vi "Load_Window_Bounds.vi"(4 "Open at mouse position?":bool, 5 "Open maximised?":bool, 6 "Re-entrant user message window? (F)":bool, 7 "Window Name (i.e. Key)":string, 8 "error in":errorcluster, 9 "Disable":bool, 10 "First Call":bool, 11 "Window VI's Ref":refnum<vi>) -> (0 "error out":errorcluster, 1 "Front Panel.WinBounds":T1, 2 "Window size":cluster{"Horisontal":i16, "Vertical":i16}, 3 "reference out":refnum<vi>)   [LabVIEW 2013]
uses:
  <vilib>/Utility/miscctls.llb/LVRectTypeDef.ctl
  Typedefs/Which path.ctl
  Typedefs/Window position FG states.ctl
  <vilib>/Utility/config.llb/Read Key (String).vi
  <vilib>/Utility/config.llb/NI_LVConfig.lvlib
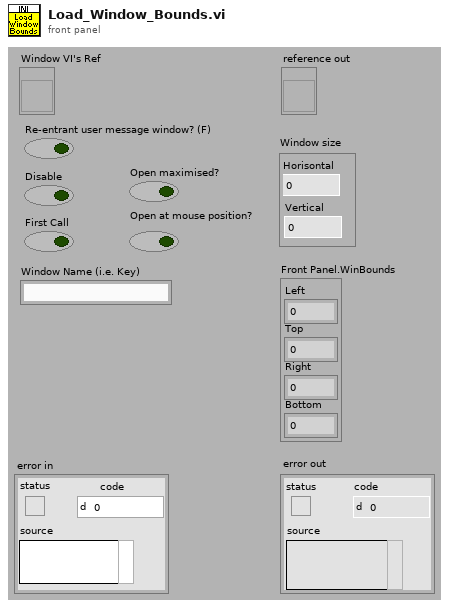
[diagram p1: front panel]
types:
  T1 = typedef "LVRectTypeDef.ctl" = cluster{"Left":i16, "Top":i16, "Right":i16, "Bottom":i16}
  T2 = enum32{"Invalid", "Standard", "Closed", "Hidden", "Minimized", "Maximized"}
  T3 = typedef "Which path.ctl" = enum16{"Configuration Files", "Calibration Files", "Images", "Setup.ini", "Loaded User profile.ini", "User's-Previous session.ini", "New user profile.ini", "Selected User profile.ini", "User profiles folder", "Power meter scaling.txt", "FOV Cal.ini"}
  T4 = typedef "Window position FG states.ctl" = enum16{"Manage", "Query", "Write"}
  T5 = typedef "NI_LVConfig.lvlib/Config Data RefNum.ctl" = refnum<k1>
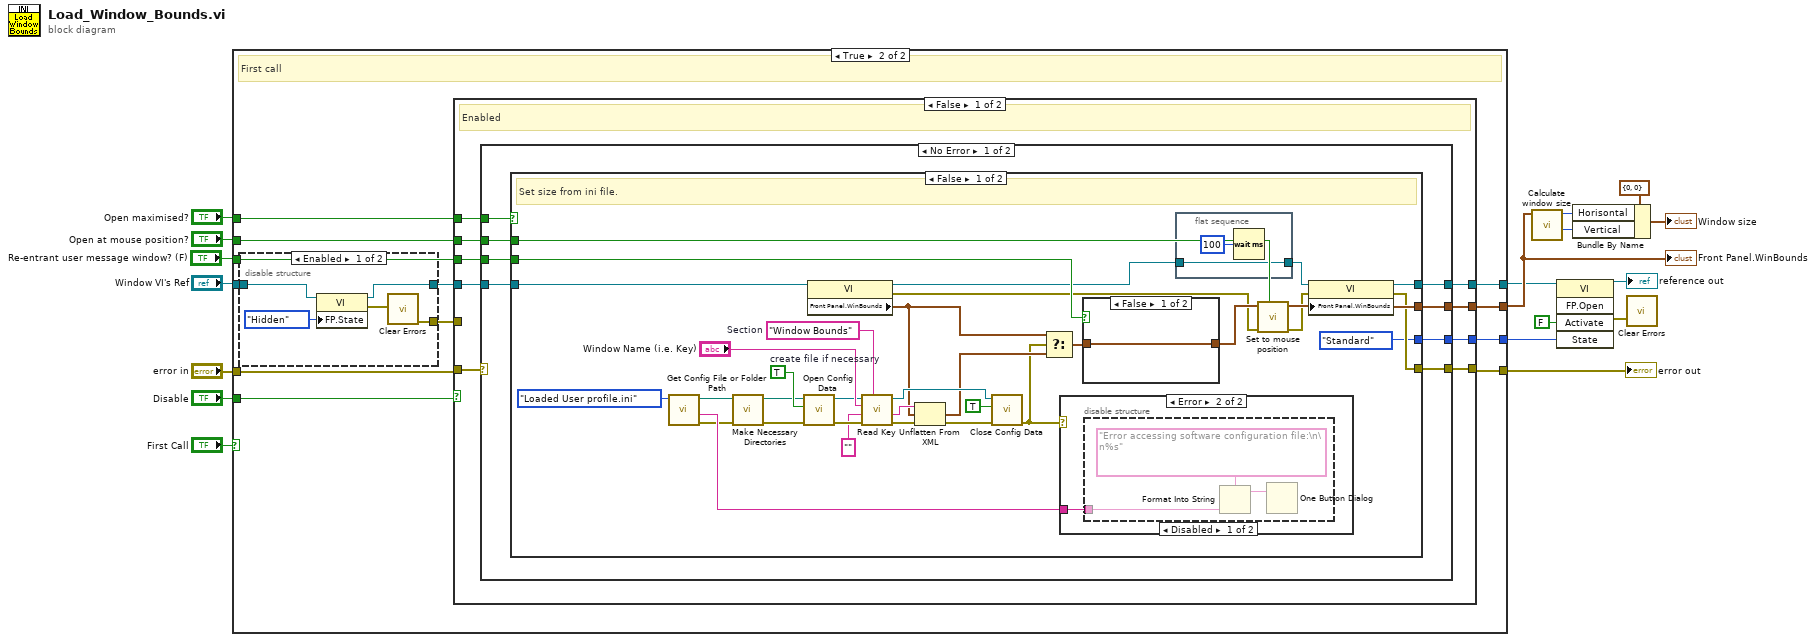
[diagram p0: block diagram]
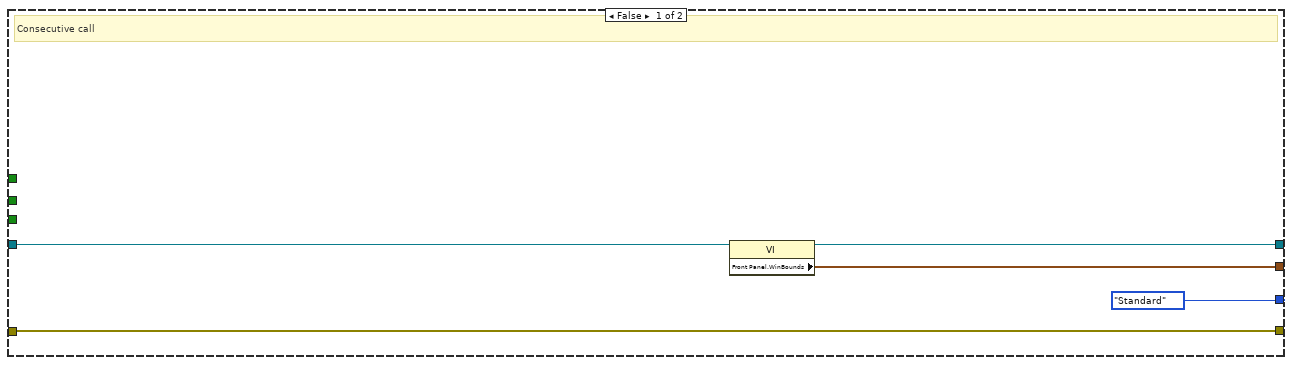
[diagram p2: hidden frame]
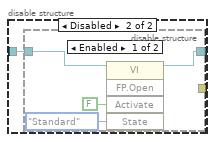
[diagram p3: hidden frame]
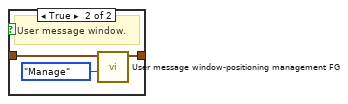
[diagram p5: hidden frame]
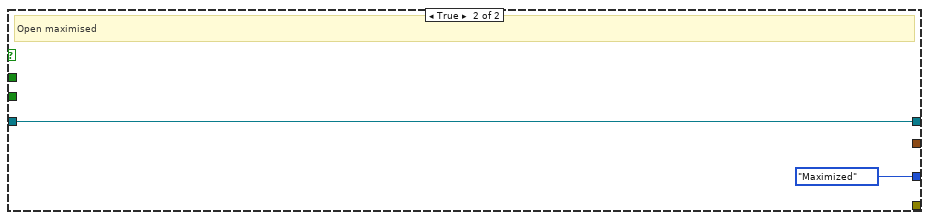
[diagram p8: hidden frame]
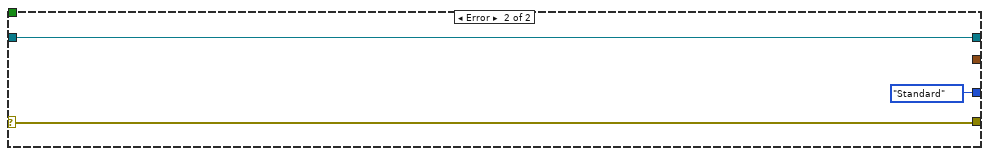
[diagram p9: hidden frame]
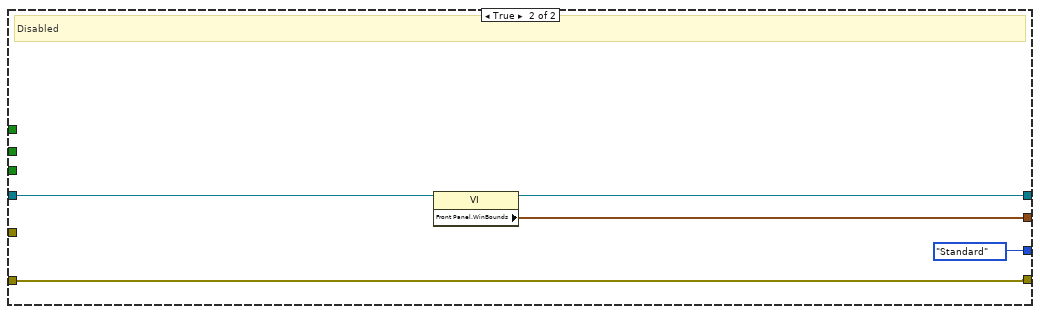
[diagram p10: hidden frame]
diagram:
  n1 = case shown="True" "First Call" {
    tunnel: "error in" -> [w23 w35]
    tunnel: "Disable" -> [_ w34]
    tunnel: "Window VI's Ref" -> [w22 w30]
    tunnel: [w21 w33] -> w1
    tunnel: [w23 w32] -> w15
    tunnel: "Re-entrant user message window? (F)" -> [_ w28]
    tunnel: [w20 w27] -> w10
    tunnel: "Open at mouse position?" -> [_ w26]
    tunnel: "Open maximised?" -> [_ w25]
    tunnel: [T2."Standard" ("Front Panel Window:State") w24] -> w3
    frame False {
      # "Consecutive call"
      n2 = property class="VI"(reference=w22) -> (reference out=w21:refnum<vi>, "Front Panel.WinBounds"=w20:T1)  [unwired: 1 in, 1 out]
    }
    frame True {
      # "First call"
      n3 = disable-structure shown="Enabled" {
        disable-tunnel: [w39 _] -> w31
        disable-tunnel: w30 -> [w38 w42]
        disable-tunnel: [w37 w41] -> w29
        frame Enabled {
          n4 = property class="VI"(reference=w38, "FP.State"=T2."Hidden" ("Front Panel Window:State")) -> (reference out=w37:refnum<vi>, error out=w40:errorcluster)  [unwired: 1 in]
          n5 = call <vilib>:"Clear Errors.vi"("error in (no error)"=w40) -> ("error out"=w39:errorcluster)  [unwired: 6 in]
        }
        frame Disabled {
          n6 = disable-structure shown="Enabled" {
            disable-tunnel: w42 -> [w46 w47]
            disable-tunnel: [w45 w47] -> w41
            frame Enabled {
              n7 = invoke class="VI" method="FP.Open"(reference=w46, "Activate"=FALSE ("Activate?"), "State"=T2."Standard") -> (reference out=w45:refnum<vi>)  [unwired: 2 in, 4 out]
            }
            frame Disabled {
            }
          }
        }
      }
      n8 = case shown="False" w34 {
        tunnel: w29 -> [w56 w115]
        tunnel: [w55 w117] -> w32
        tunnel: [w54 w114] -> w33
        tunnel: w35 -> [w53 w117]
        tunnel: w31 -> [_ _]
        tunnel: w28 -> [w52 _]
        tunnel: [w51 w116] -> w27
        tunnel: w26 -> [w50 _]
        tunnel: w25 -> [w49 _]
        tunnel: [w48 T2."Standard" ("Front Panel Window:State")] -> w24
        frame False {
          # "Enabled"
          n9 = case shown="No Error" w53 {
            selector: w53 -> [_ w112]
            tunnel: w56 -> [w64 w111]
            tunnel: [w58 w112] -> w55
            tunnel: [w63 w111] -> w54
            tunnel: w52 -> [w62 _]
            tunnel: [w61 _] -> w51
            tunnel: w50 -> [w60 _]
            tunnel: w49 -> [w59 _]
            tunnel: [w57 T2."Standard" ("Front Panel Window:State")] -> w48
            frame No Error {
              n10 = case shown="False" w59 {
                tunnel: w64 -> [w71 w108]
                tunnel: [w97 w108] -> w63
                tunnel: w62 -> [w82 _]
                tunnel: [w77 _] -> w61
                tunnel: w60 -> [w74 _]
                tunnel: [w73 _] -> w58
                tunnel: [T2."Standard" ("Front Panel Window:State") T2."Maximized" ("Front Panel Window:State")] -> w57
                frame False {
                  w85 = TRUE  # create file if necessary
                  w93 = "Window Bounds"  # Section
                  # "Set size from ini file."
                  n11 = call "Get Config File or Folder Path.vi"("Which file or folder?"=Which_path."Loaded User profile.ini" ("Which path?")) -> ("Error Out"=w65:errorcluster, "File/Folder name string"=w66:string, "File Path"=w67:path)  [unwired: 8 in]
                  n12 = call "Make Necessary Directories.vi"("error in"=w65, "Path"=w67) -> ("error out"=w95:errorcluster, "Duplicated path"=w80:path)  [unwired: 8 in]
                  n13 = call <vilib>:"Open Config Data.vi"("error in (no error)"=w95, "create file if necessary (T)"=w85, "configuration file path"=w80) -> ("error out"=w91:errorcluster, "refnum"=w92:T5)  [unwired: 6 in, 1 out]
                  n14 = property class="VI"(reference=w71) -> (reference out=w70:refnum<vi>, error out=w76:errorcluster, "Front Panel.WinBounds"=w81:T1)  [unwired: 1 in]
                  n15 = call-poly <vilib>:"Read Key.vi"("section"=w93, "error in (no error)"=w91, "default value"="" ("xml string"), "key"="Window Name (i.e. Key)", "refnum"=w92) -> ("error out"=w87:errorcluster, "value"=w88:string, "refnum out"=w90:T5)  [unwired: 3 in, 1 out]
                  n16 = Unflatten From XML(xml string=w88, type=w81, error in (no error)=w87) -> (value=w84:T1, error out=w86:errorcluster)
                  n17 = call <vilib>:"Close Config Data.vi"("error in (no error)"=w86, "write file if changed (T)"=TRUE ("write configuration file? (F)"), "refnum"=w90) -> ("error out"=w79:errorcluster)  [unwired: 7 in, 1 out]
                  n18 = Select(t=w81, s=w79, f=w84) -> (s? t:f=w83:T1)
                  n19 = case shown="Error" w79 {
                    tunnel: w66 -> [_ w104]
                    frame No Error {
                    }
                    frame Error {
                      n20 = disable-structure shown="Disabled" {
                        disable-tunnel: w104 -> [w106 _]
                        frame Disabled {
                          n21 = Format Into String(format string="Error accessing software configuration file:\n\n%s" ("message"), w106) -> (resulting string=w105:string)  [unwired: 2 in, 1 out]
                          n22 = One Button Dialog(message=w105) -> ()  [unwired: 2 out]
                        }
                        frame Enabled {
                        }
                      }
                    }
                  }
                  n23 = case shown="False" w82 {
                    tunnel: [w100 w102] -> w78
                    tunnel: w83 -> [w100 w103]
                    frame False {
                    }
                    frame True {
                      # "User message window."
                      n24 = call "User message window-positioning management FG.vi"("Function (\"Manage\")"=Window_position_FG_states."Manage" ("Function (\"Manage\")"), "Default Window position (in)"=w103) -> ("New window position to set"=w102:T1)  [unwired: 8 in, 1 out]
                    }
                  }
                  n25 = flat-sequence {
                    tunnel: w70 -> [w98]
                    tunnel: [w98] -> w69
                    frame #0 {
                      n26 = Wait (ms)(milliseconds to wait=u32 100) -> ()  [unwired: 1 out]
                    }
                  }
                  n27 = call "Set to mouse position.vi"("Open at mouse position?"=w74, "error in (no error)"=w76, "Window position to set"=w78) -> ("error out"=w75:errorcluster, "New window position to set"=w77:T1)  [unwired: 7 in]
                  n28 = property class="VI"(reference=w69, error in=w75, "Front Panel.WinBounds"=w77) -> (reference out=w97:refnum<vi>, error out=w73:errorcluster)
                }
                frame True {
                  # "Open maximised"
                }
              }
            }
            frame Error {
            }
          }
        }
        frame True {
          # "Disabled"
          n29 = property class="VI"(reference=w115) -> (reference out=w114:refnum<vi>, "Front Panel.WinBounds"=w116:T1)  [unwired: 1 in, 1 out]
        }
      }
    }
  }
  "error out" <- w15
  "Front Panel.WinBounds" <- w10
  n30 = call "Calculate window size.vi"("Window bounds"=w10) -> ("Vertical window size"=w8:i16, "Horisontal window size"=w9:i16)  [unwired: 9 in]
  n31 = invoke class="VI" method="FP.Open"(reference=w1, "Activate"=FALSE ("Activate?"), "State"=w3) -> (reference out=→"reference out":refnum<vi>, error out=w11:errorcluster)  [unwired: 2 in, 3 out]
  n32 = Bundle By Name(cluster=cluster{"Horisontal":i16, "Vertical":i16} {"Horisontal"=0, "Vertical"=0} ("Window size"), "Horisontal"=w9, "Vertical"=w8) -> (→"Window size":cluster{"Horisontal":i16, "Vertical":i16})
  n33 = call <vilib>:"Clear Errors.vi"("error in (no error)"=w11) -> ()  [unwired: 6 in, 1 out]
